vi "Position Accept Button.vi"(8 "error in (no error)":errorcluster, 10 "Title String":refnum<vi>, 11 "Accept Button":refnum<vi>) -> (0 "error out":errorcluster)   [LabVIEW 2014]
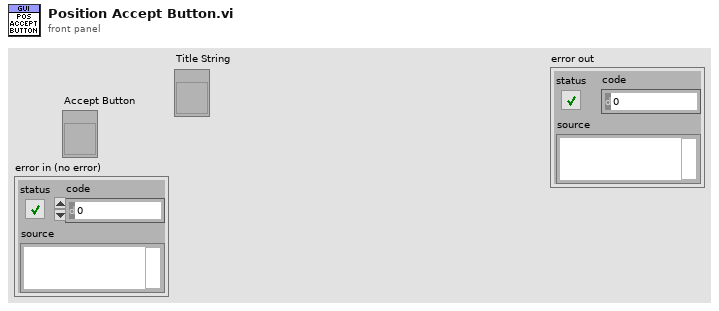
[diagram p1: front panel]
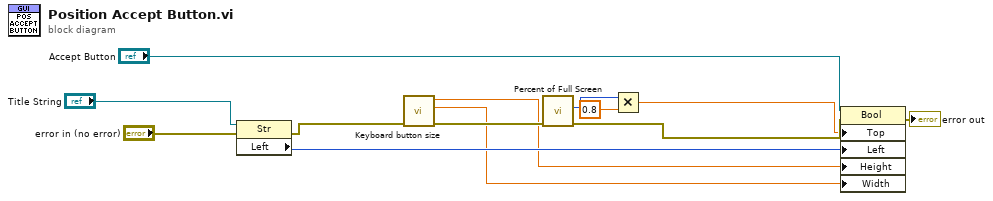
[diagram p0: block diagram]
diagram:
  n1 = property class="Str"(reference="Title String", error in="error in (no error)") -> (error out=w8:errorcluster, "Left"=w3:i32)  [unwired: 1 out]
  n2 = call "Keyboard button size.vi"("error in (no error)"=w8) -> ("error out"=w7:errorcluster, "Key Width"=w1:dbl, "Key Height"=w2:dbl)  [unwired: 7 in, 1 out]
  n3 = call "Percent of Full Screen.vi"("error in (no error)"=w7) -> ("error out"=w13:errorcluster, "Bottom"=w6:i16)  [unwired: 8 in, 1 out]
  n4 = Multiply(x=w6, y=0.8) -> (x*y=w4:dbl)
  n5 = property class="Bool"(reference="Accept Button", error in=w13, "Top"=w4, "Left"=w3, "Height"=w2, "Width"=w1) -> (error out=→"error out":errorcluster)  [unwired: 1 out]
